vi "Create.vi"(8 "error in (no error)":errorcluster, 10 "Remote Messaging":refnum<class "MessageQ.lvclass">) -> (0 "error out":errorcluster, 3 "Vecto Message Bridge out":refnum<class "Vecto Message Bridge.lvclass">)   [LabVIEW 2020, in "Volatus.lvlib" / "Vecto Message Bridge.lvclass"]
uses:
  Vecto Message Bridge.lvclass
  Vecto Message Bridge.lvclass/Vecto Message Bridge.ctl
  MessageQ/MessageQ.lvclass
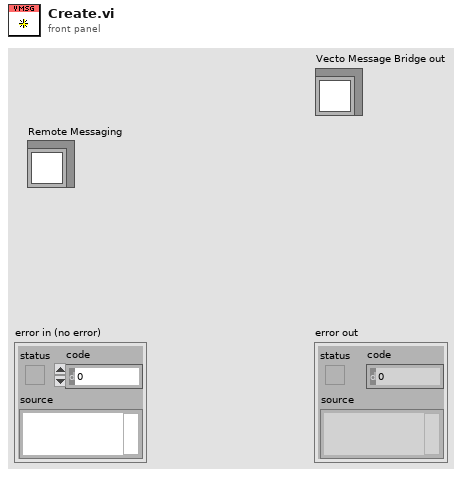
[diagram p1: front panel]
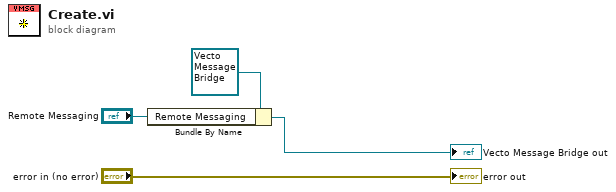
[diagram p0: block diagram]
diagram:
  n1 = Bundle By Name(cluster=refnum<class "Vecto Message Bridge.lvclass"> refnum ("Vecto Message Bridge in"), "Remote Messaging"="Remote Messaging") -> (→"Vecto Message Bridge out":refnum<class "Vecto Message Bridge.lvclass">)
  "error out" <- "error in (no error)"
